vi "Xeryon serial driver.vi"() -> ()   [LabVIEW 2019]
uses:
  <vilib>/Utility/error.llb/DialogType.ctl
  <vilib>/Instr/_visa.llb/VISA Configure Serial Port (Instr).vi
panel:
  out "COM-port":string
  in  "Send custom command":bool
  in  "Custom command":string caption="Send custom command :"
  in  "Close":bool
  out "Receive history :":string
  out "Detected stages :":i32(listbox)
  out "Send history :":i32(listbox)
  # "Xeryon Serial Driver"
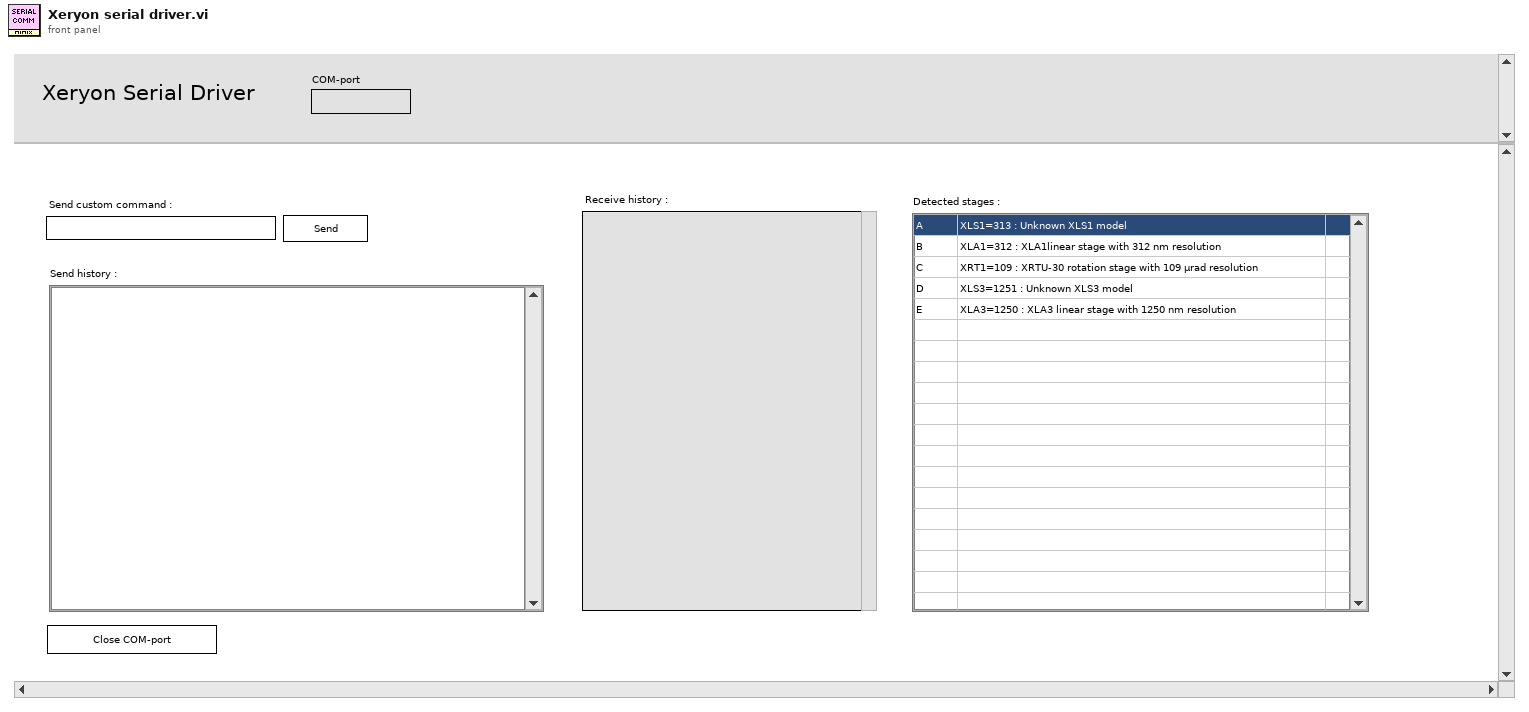
[diagram p1: front panel]
types:
  T1 = enum16{"Init", "Set stage data", "Update position", "Get"}
  T2 = typedef "Xeryon serial command.ctl" = cluster{"Command":enum16{"Send serial data", "Exit"}, "Data to send":string}
  T3 = typedef "Serial parameters.ctl" = enum16{"Serial number", "Software number", "Type of stage", "Status", "Frequency", "Encoder position", "Desired position", "Info", "Phase correction", "Timestamp", "Proportional control factor", "Sync", "XRT1", "XRT3", "XRTA", "XLS1", "XLS3", "XLA1", "XLA3"}
  T4 = cluster{"Parameters out":T3[], "Values out":i32[], "Stage type":string, "Stage letter":string}[]
  T5 = typedef "DialogType.ctl" = u16
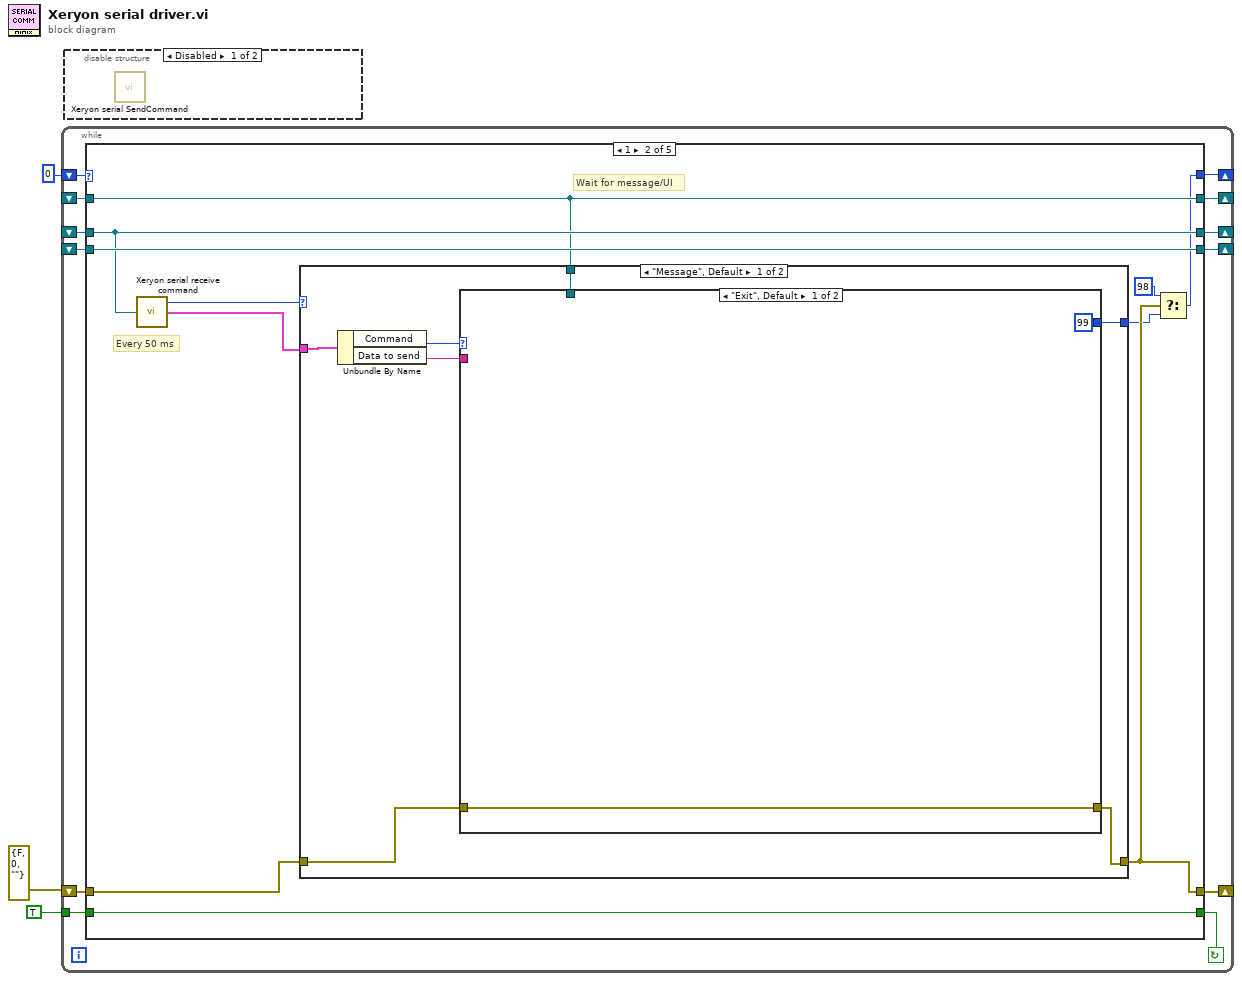
[diagram p0: block diagram]
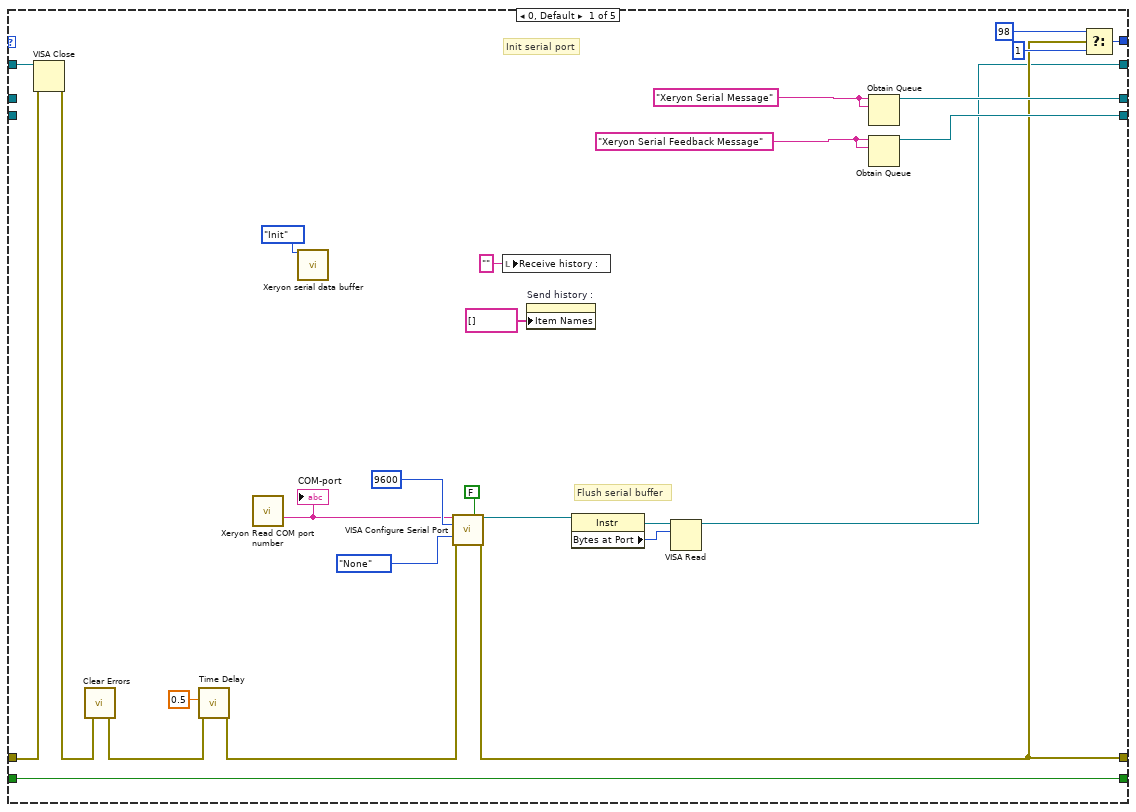
[diagram p3: hidden frame]
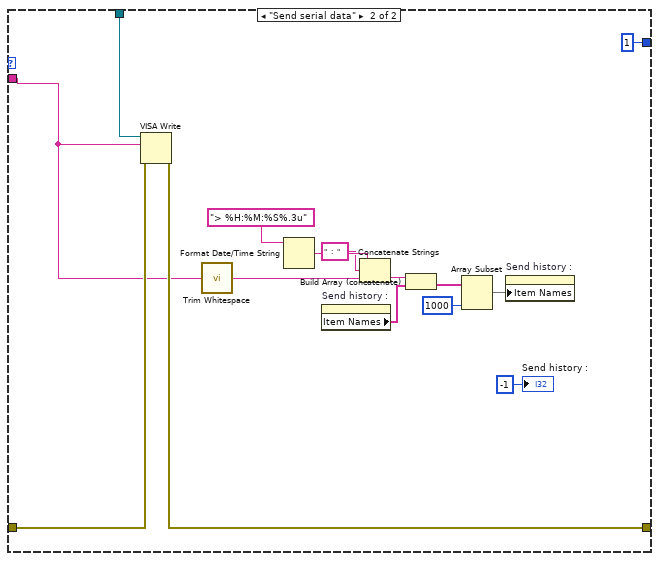
[diagram p4: hidden frame]
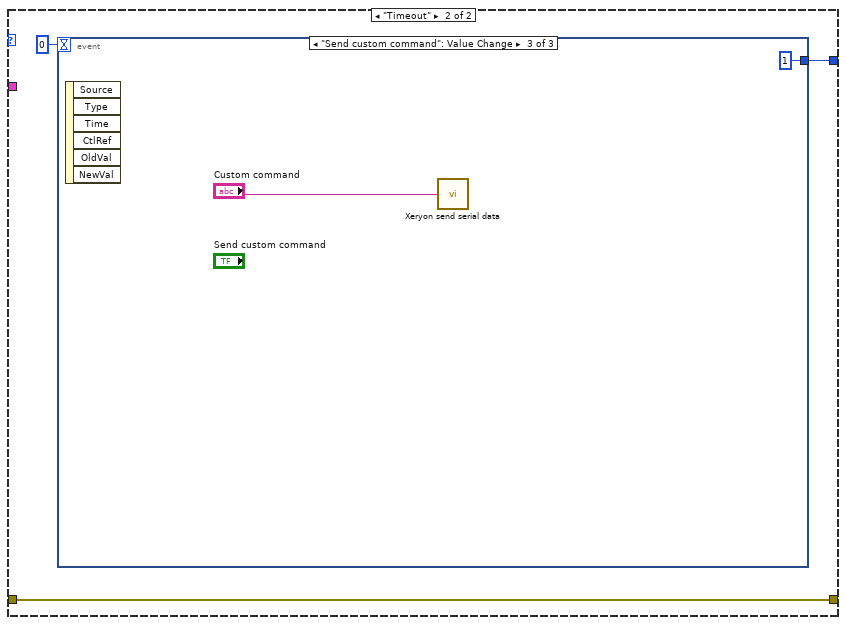
[diagram p5: hidden frame]
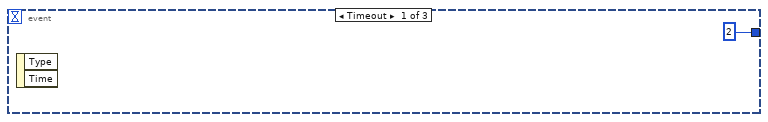
[diagram p6: hidden frame]
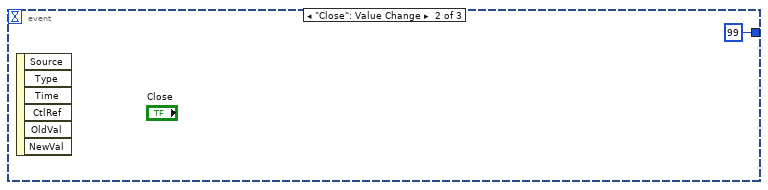
[diagram p7: hidden frame]
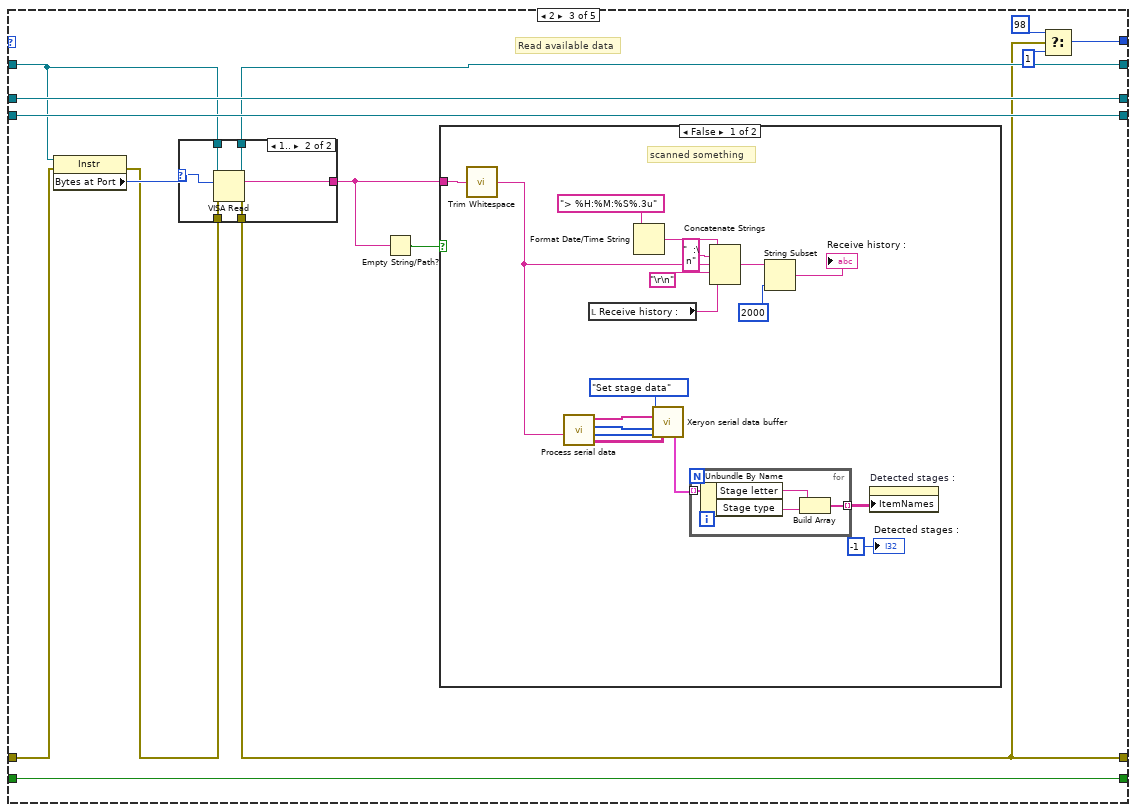
[diagram p8: hidden frame]
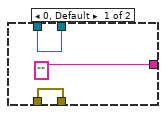
[diagram p9: hidden frame]
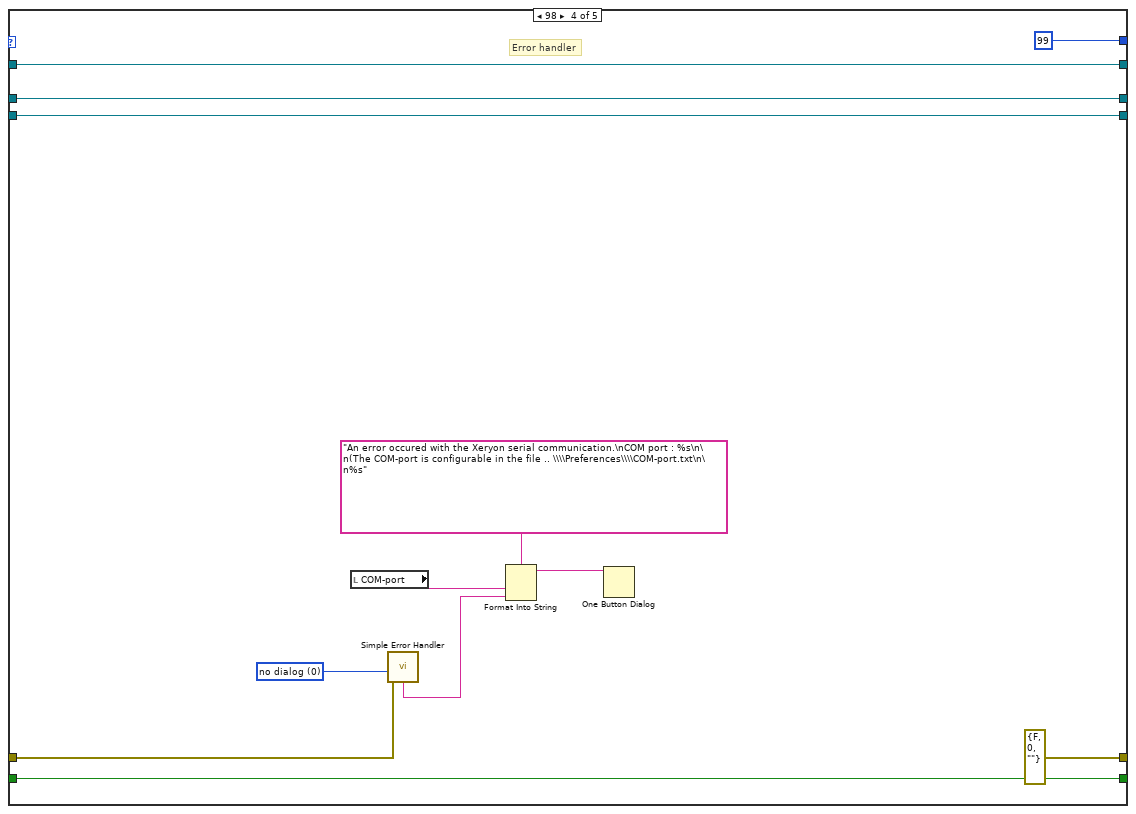
[diagram p11: hidden frame]
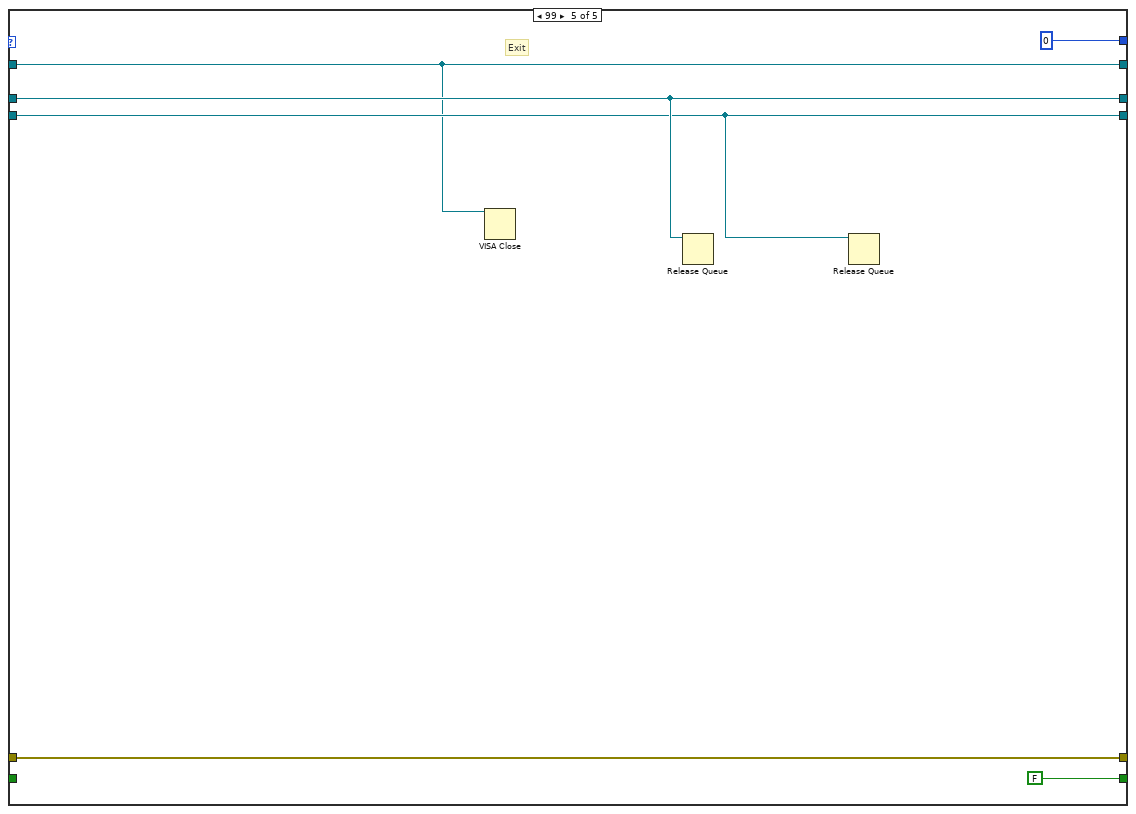
[diagram p12: hidden frame]
diagram:
  n1 = while {
    shift-right: [w9] -> _
    shift-left: 0 -> [w15]
    shift-right: [w11] -> _
    shift-left: errorcluster {"status"=FALSE, "code"=0, "source"=""} ("error in") -> [w14]
    tunnel: TRUE -> [w13]
    shift-right: [w10] -> _
    shift-left: _ -> [w8]
    shift-right: [w7] -> _
    shift-left: _ -> [w4]
    shift-right: [w6] -> _
    shift-left: _ -> [w5]
    stop <- w12 continue-if-true
    n2 = case shown="1" w15 {
      tunnel: w14 -> [w31 w47 w94 w133 w145]
      tunnel: [w41 w51 w95 w138 FALSE] -> w12
      tunnel: w13 -> [w41 w51 w95 w138 _]
      tunnel: [w33 w45 w86 errorcluster {"status"=FALSE, "code"=0, "source"=""} ("error in") w145] -> w11
      tunnel: [w26 w46 w88 w140 w141] -> w10
      tunnel: [w40 w42 w91 99 0] -> w9
      tunnel: w8 -> [w32 w46 w89 w140 w141]
      tunnel: [w37 w48 w96 w137 w143] -> w7
      tunnel: [w36 w52 w97 w136 w142] -> w6
      tunnel: w5 -> [_ w52 w97 w136 w142]
      tunnel: w4 -> [_ w48 w96 w137 w143]
      frame 0, Default {
        w21 = "Xeryon Serial Feedback Message" ("name (unnamed)")
        w22 = "Xeryon Serial Message" ("name (unnamed)")
        # "Flush serial buffer"
        # "Init serial port"
        n3 = VISA Close(VISA resource name=w32, error in (no error)=w31) -> (error out=w30:errorcluster)
        n4 = call <vilib>:"Clear Errors.vi"("error in (no error)"=w30) -> ("error out"=w25:errorcluster)  [unwired: 5 in, 1 out]
        n5 = call "Time Delay"("error in (no error)"=w25, "Delay Time (s)"=0.5) -> ("error out"=w24:errorcluster)  [unwired: 9 in]
        n6 = call "Xeryon Read COM port number.vi"() -> ("COM-port"=w16:string)  [unwired: 5 in]
        "COM-port" <- w16
        n7 = call "Xeryon serial data buffer.vi"("Mode"=T1."Init") -> ()  [unwired: 8 in, 7 out]
        n8 = call-poly "VISA Configure Serial Port"("VISA resource name"=w16, "Enable Termination\nChar (T)"=FALSE ("Enable Termination\nChar (T)"), "baud rate (9600)"=u32 9600, "parity (0:none)"=enum16{"None", "Odd", "Even", "Mark", "Space"}."None", "error in (no error)"=w24) -> ("VISA resource name out"=w27:refnum<visa-resource-name>, "error out"=w33:errorcluster)  [unwired: 9 in]
        n9 = local write "Receive history :"("" ("Receive history :")) -> ()
        n10 = property on="Send history :" class="LstBox (strict)"("Item Names"=string[] []) -> ()  [unwired: 2 in, 2 out]
        n11 = property class="Instr"(reference=w27) -> (reference out=w29:refnum<visa-resource-name>, "Bytes at Port"=w28:u32)  [unwired: 1 in, 1 out]
        n12 = VISA Read(VISA resource name=w29, byte count=w28) -> (VISA resource name out=w26:refnum<visa-resource-name>)  [unwired: 1 in, 3 out]
        n13 = Obtain Queue(name (unnamed)=w22, element data type=w22) -> (queue out=w37:refnum<queue>)  [unwired: 3 in, 2 out]
        n14 = Obtain Queue(name (unnamed)=w21, element data type=w21) -> (queue out=w36:refnum<queue>)  [unwired: 3 in, 2 out]
        n15 = Select(t=98, s=w33, f=1) -> (s? t:f=w40:i32)
      }
      frame 1 {
        # "Every 50 ms"
        # "Wait for message/UI"
        n16 = call "Xeryon serial receive command.vi"("queue out"=w48) -> ("Type"=w50:enum16{"Message", "Timeout"}, "Serial Message"=w49:T2)  [unwired: 1 out]
        n17 = case shown="\"Message\", Default" w50 {
          tunnel: w49 -> [w59 _]
          tunnel: [w56 w79] -> w44
          tunnel: [w54 w78] -> w45
          tunnel: w47 -> [w55 w78]
          tunnel: w46 -> [w53 _]
          frame "Message", Default {
            n18 = Unbundle By Name(w59) -> ("Command"=w58:enum16{"Send serial data", "Exit"}, "Data to send"=w57:string)
            n19 = case shown="\"Exit\", Default" w58 {
              tunnel: w57 -> [_ w64]
              tunnel: [99 1] -> w56
              tunnel: [w60 w73] -> w54
              tunnel: w55 -> [w60 w74]
              tunnel: w53 -> [_ w75]
              frame "Exit", Default {
              }
              frame "Send serial data" {
                n20 = VISA Write(VISA resource name=w75, write buffer=w64, error in (no error)=w74) -> (error out=w73:errorcluster)  [unwired: 2 out]
                n21 = call <vilib>:"Trim Whitespace.vi"("string"=w64) -> ("trimmed string"=w63:string)  [unwired: 1 in]
                n22 = Format Date/Time String(time format string (%c)="> %H:%M:%S%.3u") -> (date/time string=w72:string)  [unwired: 2 out]
                n23 = property on="Send history :" class="LstBox (strict)"() -> ("Item Names"=w69:string[])  [unwired: 2 in, 2 out]
                n24 = Concatenate Strings(w72, "  :  " ("string"), w63) -> (w71:string)
                n25 = Build Array (concatenate)(w71, w69) -> (w70:string[])
                n26 = Array Subset(array=w70, length=1000) -> (w68:string[])  [unwired: 1 in]
                n27 = property on="Send history :" class="LstBox (strict)"("Item Names"=w68) -> ()  [unwired: 2 in, 2 out]
                "Send history :" <- -1 ("Send history :")
              }
            }
          }
          frame "Timeout" {
            n28 = event shown="[2] \"Send custom command\": Value Change" {
              selector: _ -> [_ _ _]
              dyn-events: _ -> [_ _ _]
              timeout: 0 -> [_ _ _]
              tunnel: [2 99 1] -> w79
              event Timeout {
                n29 = event-data() -> ()  [unwired: 3 out]
              }
              event "Close": Value Change {
                n30 = event-data() -> ()  [unwired: 7 out]
              }
              event "Send custom command": Value Change {
                n31 = event-data() -> ()  [unwired: 7 out]
                n32 = call "Xeryon send serial data.vi"("Data to send"="Custom command") -> ()  [unwired: 5 in]
              }
            }
          }
        }
        n33 = Select(t=98, s=w45, f=w44) -> (s? t:f=w42:i32)
      }
      frame 2 {
        # "Read available data"
        n34 = property class="Instr"(reference=w89, error in=w94) -> (error out=w87:errorcluster, "Bytes at Port"=w90:u32)  [unwired: 1 out]
        n35 = case shown="1.." w90 {
          selector: w90 -> [_ w101]
          tunnel: w89 -> [w100 w106]
          tunnel: [w100 w105] -> w88
          tunnel: ["" w104] -> w85
          tunnel: w87 -> [w98 w103]
          tunnel: [w98 w102] -> w86
          frame 0, Default {
          }
          frame 1.. {
            n36 = VISA Read(VISA resource name=w106, byte count=w101, error in (no error)=w103) -> (VISA resource name out=w105:refnum<visa-resource-name>, read buffer=w104:string, error out=w102:errorcluster)  [unwired: 1 out]
          }
        }
        n37 = Empty String/Path?(string/path=w85) -> (empty?=w84:bool)
        n38 = case shown="False" w84 {
          tunnel: w85 -> [w121 _]
          frame False {
            # "scanned something"
            n39 = call <vilib>:"Trim Whitespace.vi"("string"=w121) -> ("trimmed string"=w120:string)  [unwired: 1 in]
            n40 = call "Process serial data.vi"("Data in"=w120) -> ("Stage types"=w116:string[][], "Values"=w117:i32[], "Parameters"=w118:T3[], "Drive letters"=w119:string[])  [unwired: 3 in]
            n41 = local read "Receive history :"() -> (w111:string)
            n42 = Format Date/Time String(time format string (%c)="> %H:%M:%S%.3u") -> (date/time string=w124:string)  [unwired: 2 out]
            n43 = call "Xeryon serial data buffer.vi"("Mode"=T1."Set stage data", "Stage types in"=w116, "Drive letters in"=w119, "Parameters in"=w118, "Values in"=w117) -> ("Stage data"=w113:T4)  [unwired: 4 in, 6 out]
            n44 = for {
              tunnel: w113 -> [w127] mode=indexing
              tunnel: [w128] -> w114 mode=indexing
              n45 = Unbundle By Name(w127) -> ("Stage letter"=w126:string, "Stage type"=w125:string)
              n46 = Build Array(w126, w125) -> (w128:string[])
            }
            n47 = Concatenate Strings(w124, "  :\n" ("string"), w120, "\r\n", w111) -> (w109:string)
            n48 = String Subset(string=w109, length (rest)=2000 ("length (rest)")) -> (substring=→"Receive history :":string)  [unwired: 1 in]
            n49 = property on="Detected stages :" class="MCListbox (strict)"("ItemNames"=w114) -> ()  [unwired: 2 in, 2 out]
            "Detected stages :" <- -1 ("Detected stages :")
          }
          frame True {
            # "no data"
          }
        }
        n50 = Select(t=98, s=w86, f=1 ("t")) -> (s? t:f=w91:i32)
      }
      frame 98 {
        w132 = T5 0 items=["no dialog", "OK message", "continue or stop message", "OK message + warnings", "continue/stop + warnings"] ("type of dialog (OK msg:1)")
        # "Error handler"
        n51 = local read "COM-port"() -> (w129:string)
        n52 = call <vilib>:"Simple Error Handler.vi"("type of dialog (OK msg:1)"=w132, "error in (no error)"=w133) -> ("message"=w131:string)  [unwired: 3 in, 4 out]
        n53 = Format Into String(format string="An error occured with the Xeryon serial communication.\nCOM port : %s\n\n(The COM-port is configurable in the file .. \\\\Preferences\\\\COM-port.txt\n\n%s" ("Algemene omschrijving"), w129, w131) -> (resulting string=w130:string)  [unwired: 2 in, 1 out]
        n54 = One Button Dialog(message=w130) -> ()  [unwired: 1 in, 1 out]
      }
      frame 99 {
        # "Exit"
        n55 = VISA Close(VISA resource name=w141) -> ()  [unwired: 1 in, 1 out]
        n56 = Release Queue(queue=w143) -> ()  [unwired: 1 in, 4 out]
        n57 = Release Queue(queue=w142) -> ()  [unwired: 1 in, 4 out]
      }
    }
  }
  n58 = disable-structure shown="Disabled" {
    frame Disabled {
      n59 = call "Xeryon serial SendCommand.vi"() -> ()  [unwired: 3 in, 3 out]
    }
    frame Enabled {
    }
  }
